vi "Draw.vi"(8 "error in (no error)":errorcluster, 9 "disable contained items?":bool, 10 "IB_Tree":refnum<class "IB_Tree.lvclass">, 11 "IB_TreeItem in":refnum<class "IB_Tree_Item.lvclass">) -> (0 "error out":errorcluster, 3 "IB_TreeItem out":refnum<class "IB_Tree_Item.lvclass">)   [LabVIEW 2020, in "IB_Tree_Item.lvclass"]
uses:
  <vilib>/AppBuilder/IB_Classes/Tree_Item/IB_Tree_Item.lvclass
  <vilib>/AppBuilder/IB_Classes/Tree_Item/IB_Tree_Item.lvclass/IB_Tree_Item.ctl
  <vilib>/AppBuilder/IB_Classes/Tree/IB_Tree.lvclass
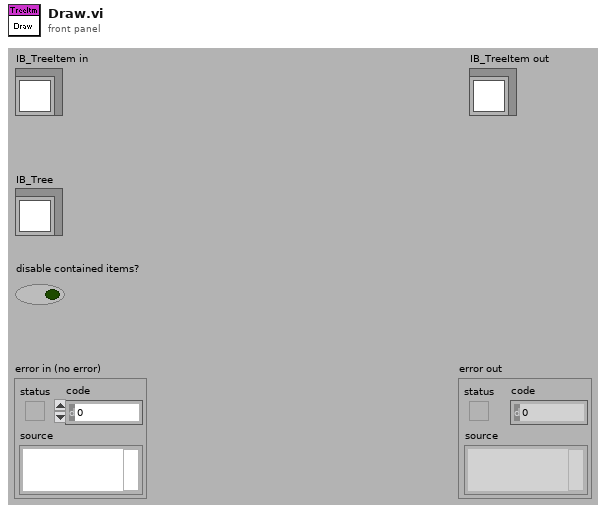
[diagram p1: front panel]
types:
  T1 = typedef "IB_Tree_Item.ctl" = cluster{"symbol index":i32, "child tag":string, "parentTag":string, "left cell name":string}
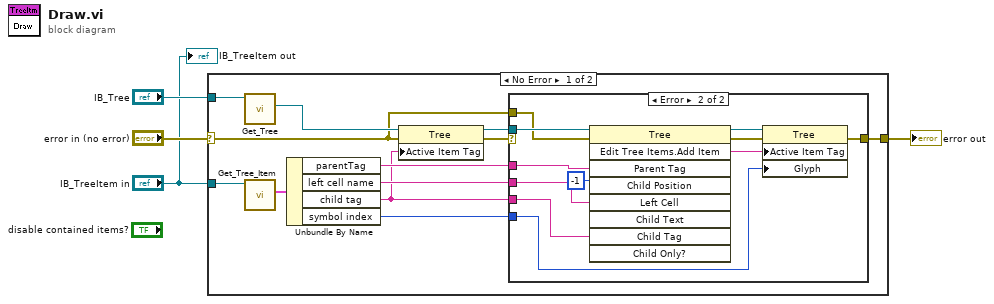
[diagram p0: block diagram]
diagram:
  n1 = case shown="No Error" "error in (no error)" {
    selector: "error in (no error)" -> [w5 w29]
    tunnel: "IB_TreeItem in" -> [w14 _]
    tunnel: [w16 w29] -> w4
    tunnel: "IB_Tree" -> [w10 _]
    frame No Error {
      n2 = call <vilib>:"Get_Tree.vi"("IB_Tree in"=w10) -> ("ctl"=w9:refnum<vi>)  [unwired: 1 in, 9 out]
      n3 = call <vilib>:"Get_Tree_Item.vi"("IB_TreeItem in"=w14) -> ("data"=w13:T1)  [unwired: 1 in, 9 out]
      n4 = Unbundle By Name(w13) -> ("parentTag"=w12:string, "left cell name"=w11:string, "child tag"=w6:string, "symbol index"=w15:i32)
      n5 = property class="Tree"(reference=w9, error in=w5, "Active Item Tag"=w6) -> (reference out=w8:refnum<vi>, error out=w7:errorcluster)
      n6 = case shown="Error" w7 {
        selector: w7 -> [w17 _]
        tunnel: [w17 w26] -> w16
        tunnel: w15 -> [_ w24]
        tunnel: w6 -> [_ w23]
        tunnel: w12 -> [_ w22]
        tunnel: w11 -> [_ w21]
        tunnel: w8 -> [_ w20]
        tunnel: w5 -> [_ w19]
        frame No Error {
        }
        frame Error {
          n7 = invoke class="Tree" method="Edit Tree Items.Add Item"(reference=w20, error in=w19, "Parent Tag"=w22, "Child Position"=-1, "Left Cell"=w21, "Child Tag"=w23) -> (reference out=w28:refnum<vi>, error out=w27:errorcluster, "Edit Tree Items:Add Item"=w25:string)  [unwired: 3 in, 6 out]
          n8 = property class="Tree"(reference=w28, error in=w27, "Active Item Tag"=w25, "Glyph"=w24) -> (error out=w26:errorcluster)  [unwired: 1 out]
        }
      }
    }
    frame Error {
    }
  }
  "error out" <- w4
  "IB_TreeItem out" <- "IB_TreeItem in"
